vi "运维调试_总磷总氮.vi"() -> ()   [LabVIEW 2016, in "斯坦道总氮V2.lvlib"]
uses:
  <vilib>/Utility/miscctls.llb/LVPointTypeDef.ctl
  <vilib>/Plasmionique/MB Master/MB_Master/MB_Master.lvclass
  <vilib>/ptbypt/NI_PtbyPt.lvlib
panel:
  out "步骤":i32
  in  "周期设置":bool
  in  "流程写入":bool
  in  "修改系列号":bool
  out "权限等级":string
  out "总步数":i32
  out "滑动杆":u8(slide) caption="测试进度" scale=0.0..100.0
  in  "关闭心跳包":bool
  in  "仪器校准":bool
  in  "参数查询":bool
  out "简易步骤名称":string
  in  "温度曲线":bool
  in  "启动参数设置":bool
  out "固件版本号":string
  out "模块版本号":string
  out "注射器温度":sgl
  out "消解温度":sgl
  out "ADC":sgl
  out "F3":sgl format="%#.6f"
  out "F2":sgl format="%#.6f"
  out "F1":sgl format="%#.6f"
  out "F0":sgl format="%#.6f"
  out "运行状态":T1 {"数据时间:" format="%<%y/%m/%d %H:%M:%S>T"; "仪器时间:" format="%<%y/%m/%d %H:%M:%S>T"}
  in  "单选按钮":T2(radio)=enum."总氮"
  in  "布尔":bool
  out "字符串 2":string
  in  "数组":string[](array[string])
  in  "返回":bool
  in  "参数设置":bool
  out "集成报警信息":string
  in  "停止":bool
  in  "手动启动":bool
  in  "调试":bool
  out "多列列表框":i32(listbox)
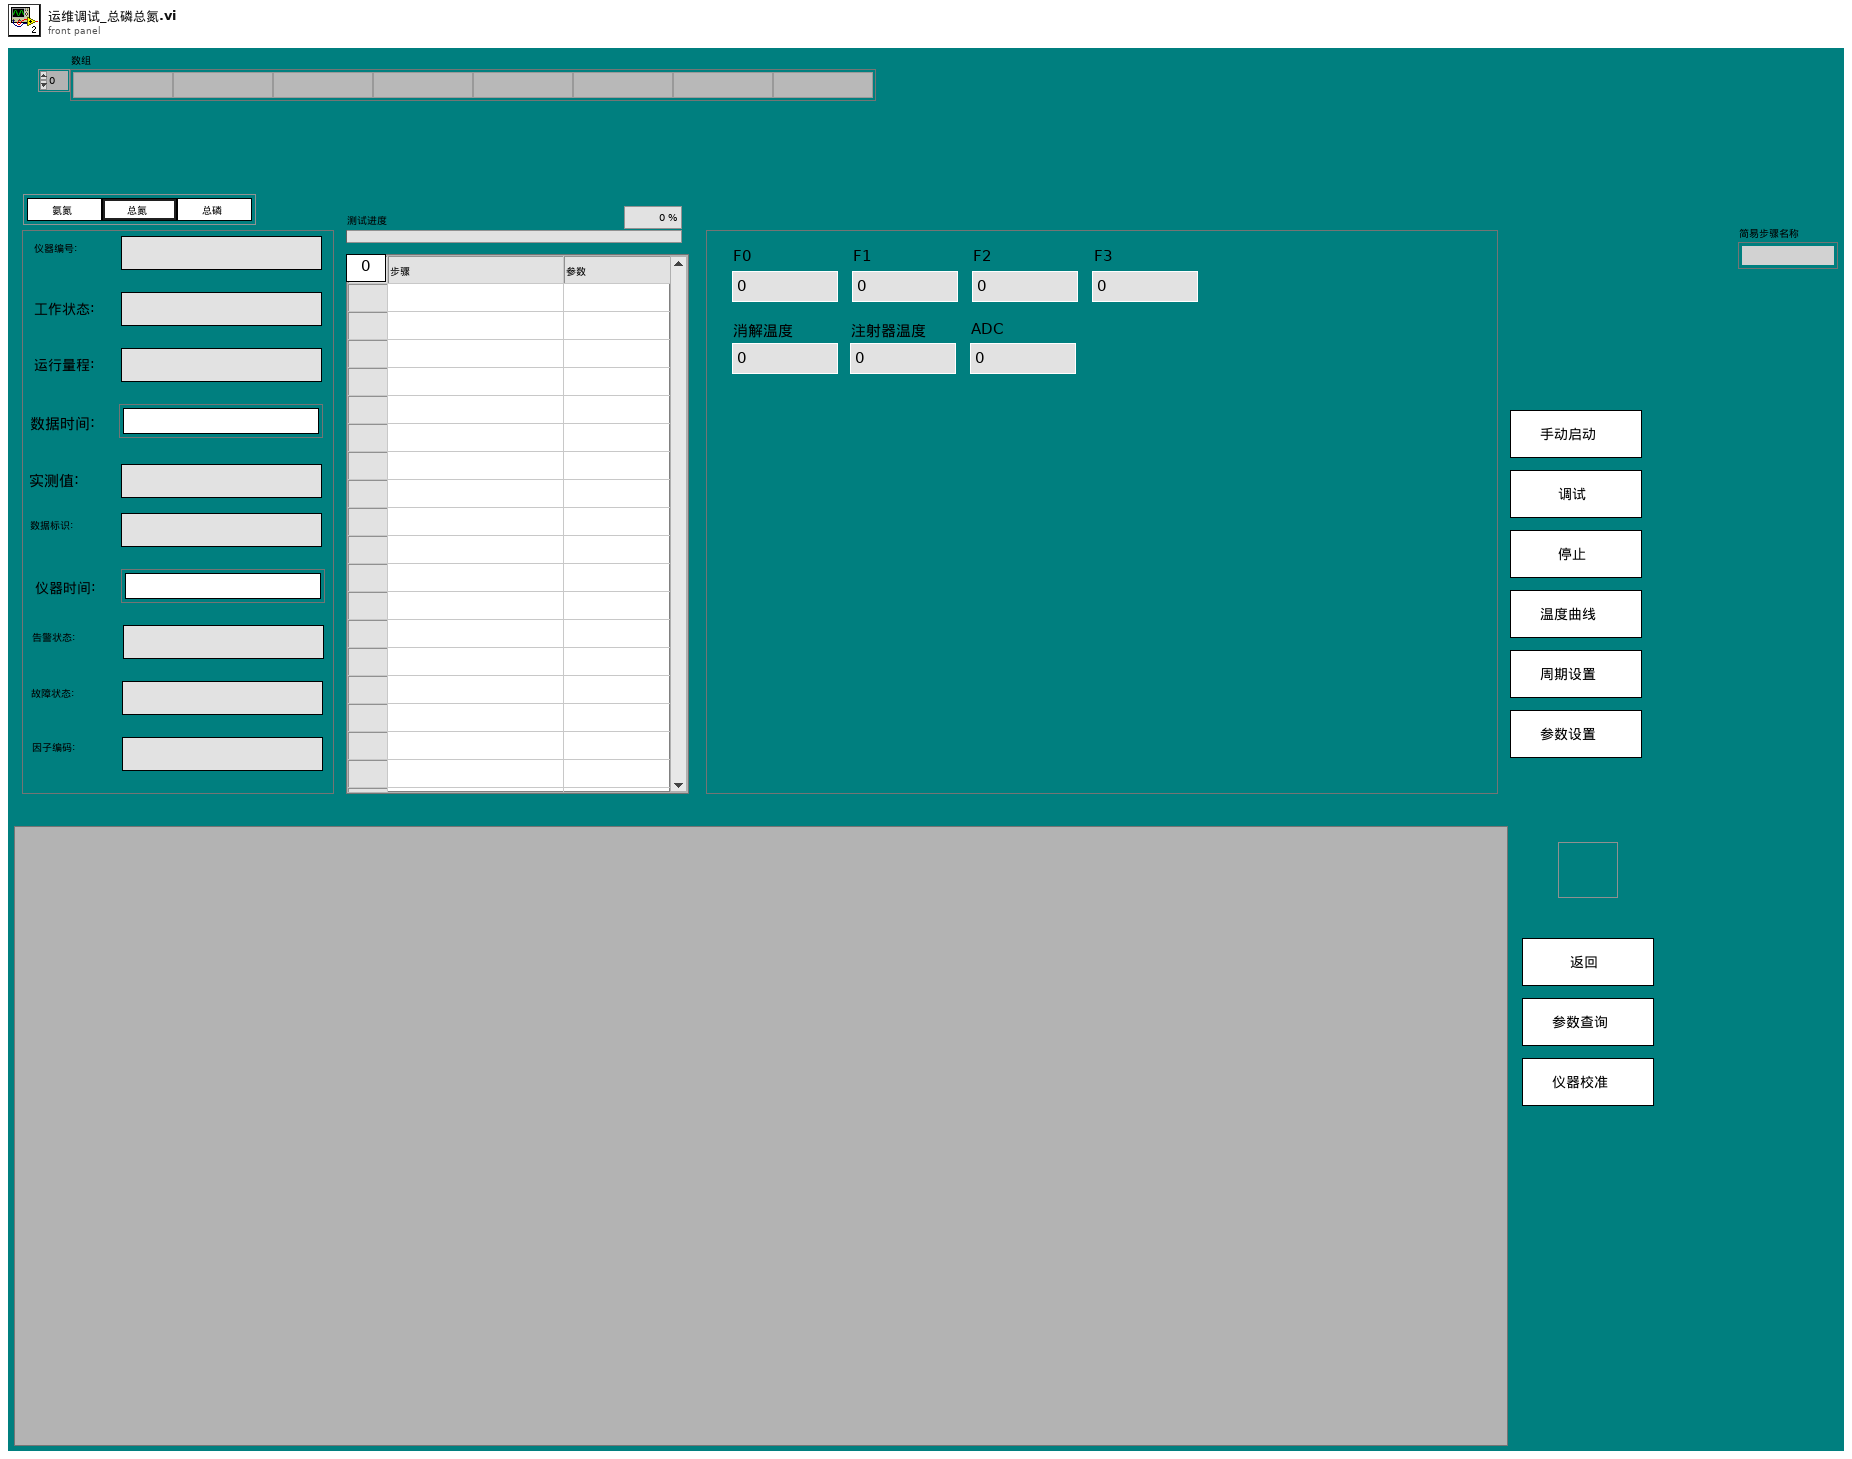
[diagram p1: front panel]
types:
  T1 = cluster{"仪器编号:":string, "工作状态:":string, "运行量程: ":string, "数据时间:":timestamp, "实测值:":string, "数据标识: ":string, "仪器时间:":timestamp, "告警状态: ":string, "故障状态:  ":string, "因子编码:":string}
  T2 = enum32{"COD", "氨氮", "总氮", "总磷", "磷酸盐", "硝氮", "亚硝氮", "硅酸盐", "硫化物"}
  T3 = cluster{"Major":u16, "Minor":u16, "Fix":u16, "Build":u16}
  T4 = typedef "LVPointTypeDef.ctl" = cluster{"Horizontal":i16, "Vertical":i16}
  T5 = cluster{"系统时间":timestamp, "工作状态":u16, "测量模式":enum16{"待机", "连续模式", "周期模式", "定点模式", "受控模式", "手动模式"}, "告警代码":u16, "故障代码":u16, "日志代码":u16, "软件版本":u16, "F0":sgl, "F1":sgl, "F2":sgl, "F3":sgl, "T":sgl, "H":sgl, "id":u16, "flowid":u16, "量程":u16, "总磷控温温度1":sgl, "营养盐控温温度2":sgl, "ADC":sgl}
  T6 = cluster{"因子编码":u32, "单位":u16, "标样参考值":sgl, "水样数据时间":timestamp, "水样实测值":sgl, "水样数据标识":string, "标样数据时间":timestamp, "标样实测值":sgl, "标样数据标识":string, "空白数据时间":timestamp, "空白实测值":sgl, "空白数据标识":string, "零点核查数据时间":timestamp, "零点核查实测值":sgl, "零点核查数据标识":string, "跨度核查数据时间":timestamp, "跨度核查实测值":sgl, "跨度核查数据标识":string, "加标回收数据时间":timestamp, "加标回收实测值":sgl, "加标回收数据标识":string, "平行样数据时间":timestamp, "平行样实测值":sgl, "平行样数据标识":string, "F0":sgl, "F1":sgl, "F2":sgl, "F3":sgl, "F4":sgl, "F5":sgl, "F6":sgl, "F7":sgl, "温度":sgl, "湿度":sgl, "X值":sgl, "fidrange":u16}[]
  T7 = cluster{"因子编码":u32, "单位":u16, "标样参考值":sgl, "水样数据时间":timestamp, "水样实测值":sgl, "水样数据标识":string, "标样数据时间":timestamp, "标样实测值":sgl, "标样数据标识":string, "空白数据时间":timestamp, "空白实测值":sgl, "空白数据标识":string, "零点核查数据时间":timestamp, "零点核查实测值":sgl, "零点核查数据标识":string, "跨度核查数据时间":timestamp, "跨度核查实测值":sgl, "跨度核查数据标识":string, "加标回收数据时间":timestamp, "加标回收实测值":sgl, "加标回收数据标识":string, "平行样数据时间":timestamp, "平行样实测值":sgl, "平行样数据标识":string, "F0":sgl, "F1":sgl, "F2":sgl, "F3":sgl, "F4":sgl, "F5":sgl, "F6":sgl, "F7":sgl, "温度":sgl, "湿度":sgl, "X值":sgl, "fidrange":u16}
  T8 = typedef "Alarm interface.lvlib/报警短信语音交互.ctl" = cluster{"参数":string, "元器件":string, "故障现象":string, "code":string, "platform_alarm_code":string, "solutionList":cluster{"reason":string, "solution":string}[]}
  T9 = typedef "TimingControl.lvlib/TimingControl.lvclass/国标控制命令.ctl" = enum16{"启动测量", "标样核查", "零点核查", "跨度核查", "空白测试", "平行样测试", "加标回收", "空白校准", "标样校准", "初始化（清洗）", "停止测试", "仪器重启", "校时", "模式设置", "测量间隔设置"}
  T10 = typedef "TimingControl.lvlib/TimingControl.lvclass/测量参数.ctl" = u16
  T11 = enum32{"Bad", "Idle", "Run top level", "Running"}
  T12 = cluster{"时间标识":timestamp, "设备":string, "日志信息":string, "流程参数":string}
  T13 = typedef "LVRowAndColumnUnsignedTypeDef.ctl" = cluster{"Row":u32, "Column":u32}
  T14 = enum16{"空闲", "水样测试", "标样核查", "零点核查", "跨度核查", "空白测试", "平行样测试", "加标回收", "空白校准", "标样校准", "初始化（清洗）"}
  T15 = cluster{"站号":u16, "量程切换":enum32{"H", "L", "AUTO"}, "控制命令":enum16{"启动测量", "标样核查", "零点核查", "跨度核查", "空白测试", "平行样测试", "加标回收", "空白校准", "标样校准", "初始化（清洗）", "停止测试", "仪器重启", "校时", "模式设置", "测量间隔设置"}, "模式设置":enum16{"待机", "连续模式", "周期模式", "定点模式", "受控模式", "手动模式"}, "测量间隔":u16}
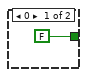
[diagram p3: hidden frame]
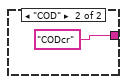
[diagram p4: hidden frame]
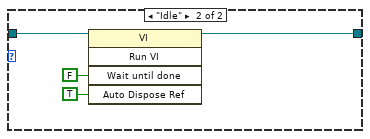
[diagram p7: hidden frame]
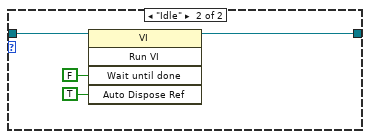
[diagram p8: hidden frame]
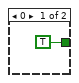
[diagram p9: hidden frame]
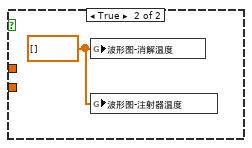
[diagram p10: hidden frame]
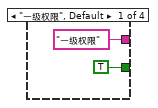
[diagram p12: hidden frame]
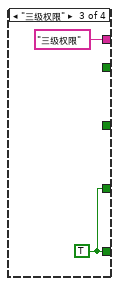
[diagram p13: hidden frame]
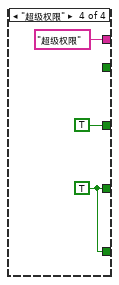
[diagram p14: hidden frame]
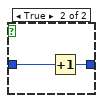
[diagram p16: hidden frame]
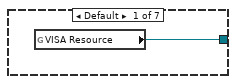
[diagram p18: hidden frame]
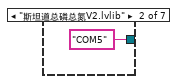
[diagram p19: hidden frame]
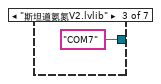
[diagram p20: hidden frame]
diagram:
  n1 = flat-sequence {
    tunnel: [w27] -> w18
    tunnel: [w26] -> w1
    tunnel: w18 -> [w38]
    tunnel: [w38] -> w4
    tunnel: w1 -> [_]
    tunnel: w4 -> [w61]
    tunnel: [w109] -> w19
    tunnel: [errorcluster {"status"=FALSE, "code"=0, "source"=""} ("错误输入（无错误）")] -> w9
    tunnel: [errorcluster {"status"=FALSE, "code"=0, "source"=""} ("错误输入（无错误）")] -> w8
    tunnel: [w106] -> w6
    tunnel: [errorcluster {"status"=FALSE, "code"=0, "source"=""} ("error out")] -> w3
    tunnel: [errorcluster {"status"=FALSE, "code"=0, "source"=""} ("错误输入（无错误）")] -> w5
    frame #0 {
      n2 = call "配置初始化.vi"() -> ("error out"=w26:errorcluster)  [unwired: 11 in]
      n3 = control-ref of="本VI"() -> (w37:refnum<vi>)
      n4 = property class="VI"(reference=w37) -> ("Library.Version"=w36:T3)  [unwired: 1 in, 2 out]
      n5 = Unbundle By Name(w36) -> ("Major"=w34:u16, "Minor"=w33:u16, "Fix"=w32:u16, "Build"=w31:u16)
      n6 = control-ref of="本VI"() -> (w28:refnum<vi>)
      n7 = Format Into String(format string="模块版本号：%d.%d.%d.%d" ("格式字符串"), w34, w33, w32, w31) -> (resulting string=→"模块版本号":string)  [unwired: 2 in, 1 out]
      n8 = property class="VI"(reference=w28) -> ("Library"=w29:refnum<vi>)  [unwired: 1 in, 2 out]
      n9 = property class="Library"(reference=w29) -> ("LocalName"=w27:string)  [unwired: 1 in, 2 out]
    }
    frame #1 {
      n10 = global read "总磷总氮断电保存全局变量.vi" "IP"() -> (w42:string)
      n11 = global read "总磷总氮断电保存全局变量.vi" "VISA Resource"() -> (w39:refnum<visa-resource-name>)
      n12 = Empty String/Path?(string/path=w42) -> (empty?=w41:bool)
      n13 = case shown="真" w41 {
        tunnel: w38 -> [_ w53]
        frame False {
        }
        frame True {
          n14 = case shown="\"斯坦道CODcrV2.lvlib\"" w53 {
            tunnel: [w54 "192.168.1.203" ("IP") "192.168.1.202" ("IP") "192.168.1.202" ("IP") "192.168.1.203" ("IP") "192.168.1.204" ("IP") "192.168.1.205" ("IP")] -> w52
            frame Default {
              n15 = global read "总磷总氮断电保存全局变量.vi" "IP"() -> (w54:string)
            }
            frame "斯坦道总磷总氮V2.lvlib" {
            }
            frame "斯坦道氨氮V2.lvlib" {
            }
            frame "斯坦道氨氮总磷V2.lvlib" {
            }
            frame "斯坦道总磷V2.lvlib" {
            }
            frame "斯坦道总氮V2.lvlib" {
            }
            frame "斯坦道CODcrV2.lvlib" {
            }
          }
          n16 = global write "总磷总氮断电保存全局变量.vi" "IP"(w52) -> ()
        }
      }
      n17 = Empty String/Path?(string/path=w39) -> (empty?=w40:bool)
      n18 = case shown="真" w40 {
        tunnel: w38 -> [_ w44]
        frame False {
        }
        frame True {
          n19 = case shown="\"斯坦道总磷V2.lvlib\"" w44 {
            tunnel: [w45 "COM5" ("IP") "COM7" ("IP") "COM7" ("IP") "COM5" ("IP") "COM10" ("IP") "COM9" ("IP")] -> w43
            frame Default {
              n20 = global read "总磷总氮断电保存全局变量.vi" "VISA Resource"() -> (w45:refnum<visa-resource-name>)
            }
            frame "斯坦道总磷总氮V2.lvlib" {
            }
            frame "斯坦道氨氮V2.lvlib" {
            }
            frame "斯坦道氨氮总磷V2.lvlib" {
            }
            frame "斯坦道总磷V2.lvlib" {
            }
            frame "斯坦道总氮V2.lvlib" {
            }
            frame "斯坦道CODcrV2.lvlib" {
            }
          }
          n21 = global write "总磷总氮断电保存全局变量.vi" "VISA Resource"(w43) -> ()
        }
      }
    }
    frame #2 {
      n22 = global read "总磷总氮断电保存全局变量.vi" "启动队列名称"() -> (w63:cluster{"String":string, "Value":u16}[])
      n23 = Empty Array?(array=w63) -> (empty?=w62:bool)
      n24 = case shown="真" w62 {
        tunnel: w61 -> [_ w64]
        frame False {
        }
        frame True {
          n25 = case shown="\"斯坦道总磷总氮V2.lvlib\"" w64 {
            frame Default {
            }
            frame "斯坦道总磷总氮V2.lvlib" {
              n26 = global write "总磷总氮断电保存全局变量.vi" "启动队列名称"(cluster{"String":string, "Value":u16}[] [{"String"="总氮", "Value"=2}, {"String"="总磷", "Value"=1}] ("启动队列名称")) -> ()
            }
            frame "斯坦道氨氮V2.lvlib" {
              n27 = global write "总磷总氮断电保存全局变量.vi" "启动队列名称"(cluster{"String":string, "Value":u16}[] [{"String"="氨氮", "Value"=3}] ("启动队列名称")) -> ()
            }
            frame "斯坦道氨氮总磷V2.lvlib" {
              n28 = global write "总磷总氮断电保存全局变量.vi" "启动队列名称"(cluster{"String":string, "Value":u16}[] [{"String"="氨氮", "Value"=3}, {"String"="总磷", "Value"=1}] ("启动队列名称")) -> ()
            }
            frame "斯坦道总磷V2.lvlib" {
              n29 = global write "总磷总氮断电保存全局变量.vi" "启动队列名称"(cluster{"String":string, "Value":u16}[] [{"String"="总磷", "Value"=1}] ("启动队列名称")) -> ()
            }
            frame "斯坦道总氮V2.lvlib" {
              n30 = global write "总磷总氮断电保存全局变量.vi" "启动队列名称"(cluster{"String":string, "Value":u16}[] [{"String"="总氮", "Value"=2}] ("启动队列名称")) -> ()
            }
            frame "斯坦道CODcrV2.lvlib" {
              n31 = global write "总磷总氮断电保存全局变量.vi" "启动队列名称"(cluster{"String":string, "Value":u16}[] [{"String"="CODcr", "Value"=22}] ("启动队列名称")) -> ()
            }
          }
        }
      }
    }
    frame #3 {
      # "初始化"
      n32 = global read "总磷总氮断电保存全局变量.vi" "流程路径"() -> (w74:path)
      n33 = global read "总磷总氮断电保存全局变量.vi" "启动队列名称"() -> (w71:cluster{"String":string, "Value":u16}[])
      n34 = call <vilib>:"Check if File or Folder Exists.vi"("path"=w74) -> ("file or folder exists?"=w78:bool)  [unwired: 8 in, 2 out]
      n35 = for {
        tunnel: w71 -> [w82] mode=indexing
        shift-right: [w81] -> w72
        shift-left: "" -> [w79]
        n36 = Unbundle By Name(w82) -> ("String"=w80:string)
        n37 = Concatenate Strings(w79, w80) -> (w81:string)
      }
      n38 = Empty String/Path?(string/path=w74) -> (empty?=w75:bool)
      n39 = Not(x=w78) -> (.not. x?=w77:bool)
      n40 = Or(x=w75, y=w77) -> (x .or. y?=w76:bool)
      n41 = global write "VAR总磷总氮全局变量.vi" "模块名称"(w72) -> ()
      n42 = case shown="真" w76 {
        frame False {
        }
        frame True {
          n43 = global read "总磷总氮断电保存全局变量.vi" "启动队列名称"() -> (w84:cluster{"String":string, "Value":u16}[])
          n44 = for {
            tunnel: w84 -> [w87] mode=indexing
            tunnel: [w86] -> w83 mode=indexing
            n45 = Unbundle By Name(w87) -> ("String"=w86:string)
          }
          n46 = call "获取默认流程路径.vi"("参数"=w83) -> ("路径"=w85:path)  [unwired: 10 in]
          n47 = global write "总磷总氮断电保存全局变量.vi" "流程路径"(w85) -> ()
        }
      }
    }
    frame #4 {
      n48 = vi-ref "总磷总氮通讯.vi"() -> (w88:refnum<vi>)
      n49 = vi-ref "总磷总氮测量数据储存.vi"() -> (w96:refnum<vi>)
      n50 = property class="VI"(reference=w88) -> ("Name"=w89:string)  [unwired: 1 in, 2 out]
      n51 = property class="VI"(reference=w96) -> ("Name"=w103:string)  [unwired: 1 in, 2 out]
      n52 = Open VI Reference(type specifier VI Refnum (for type only)=refnum<vi> refnum, vi path=w89, options=128 ("选项")) -> (vi reference=w91:refnum<vi>, error out=w93:errorcluster)  [unwired: 3 in]
      n53 = call-by-ref "开始异步调用"(reference=w91, error in=w93) -> (reference out=w95:refnum<vi>, error out=w94:errorcluster)  [unwired: 12 in]
      n54 = Open VI Reference(type specifier VI Refnum (for type only)=refnum<vi> refnum, vi path=w103, options=128 ("选项")) -> (vi reference=w101:refnum<vi>, error out=w99:errorcluster)  [unwired: 3 in]
      n55 = Close Reference(reference=w95, error in (no error)=w94) -> ()  [unwired: 1 out]
      n56 = call-by-ref "开始异步调用"(reference=w101, error in=w99) -> (reference out=w97:refnum<vi>, error out=w98:errorcluster)  [unwired: 12 in]
      n57 = Close Reference(reference=w97, error in (no error)=w98) -> ()  [unwired: 1 out]
    }
    frame #5 {
      n58 = call "配置文件路径.vi"() -> ("appended path"=w106:path)  [unwired: 11 in]
      n59 = call "设置模块队列名.vi"() -> ("Msg"=w109:string)  [unwired: 5 in]
    }
  }
  n60 = flat-sequence {
    frame #0 {
      n61 = property on="窗格" class="Pane"("Origin"=T4 {"Horizontal"=0, "Vertical"=0} ("原点")) -> ()  [unwired: 2 in, 2 out]
    }
  }
  n62 = while {
    shift-right: [w121] -> _
    shift-left: _ -> [w119]
    stop <- FALSE stop-if-true
    n63 = global write "VAR总磷总氮全局变量.vi" "最近一次工作状态"(w119) -> ()
    n64 = global read "VAR总磷总氮全局变量.vi" "状态告警区"() -> (w139:T5)
    n65 = global read "VAR总磷总氮全局变量.vi" "通讯状态"() -> (w150:bool)
    n66 = Wait (ms)(milliseconds to wait=u32 1000 ("等待时间（毫秒）")) -> ()  [unwired: 1 out]
    n67 = case shown="\"氨氮\"" "单选按钮" {
      tunnel: [22 3 2 1 4 5 6 7 8] -> w113
      frame "COD", Default {
      }
      frame "氨氮" {
      }
      frame "总氮" {
      }
      frame "总磷" {
      }
      frame "磷酸盐" {
      }
      frame "硝氮" {
      }
      frame "亚硝氮" {
      }
      frame "硅酸盐" {
      }
      frame "硫化物" {
      }
    }
    n68 = Unbundle By Name(w139) -> ("id"=w138:u16, "工作状态"=w135:u16)
    n69 = case shown="真" w150 {
      tunnel: ["通讯异常" ("集成报警信息") w244] -> w149
      frame False {
      }
      frame True {
        n70 = global read "VAR总磷总氮全局变量.vi" "状态告警区"() -> (w250:T5)
        n71 = Unbundle By Name(w250) -> ("工作状态"=w249:u16)
        n72 = feedback #1(0) -> (w247:i32)
        n73 = case shown="0" w249 {
          tunnel: w247 -> [_ w252]
          tunnel: [_ w251] -> w245
          frame 0 {
          }
          frame Default {
            n74 = Increment(x=w252) -> (x+1=w251:i32)
          }
        }
        n75 = feedback-in #1(w245) -> ()
        n76 = global read "VAR总磷总氮全局变量.vi" "测量状态"() -> (w243:string)
        n77 = Format Into String(format string="工作计时: %d 秒" ("格式字符串"), initial string=w243, w245) -> (resulting string=w244:string)  [unwired: 1 in, 1 out]
      }
    }
    "集成报警信息" <- w149
    n78 = global read "VAR总磷总氮全局变量.vi" "测量数据区数组"() -> (w124:T6)
    n79 = case shown="1, 默认" w135 {
      tunnel: w138 -> [_ w195]
      frame 0 {
      }
      frame 1, Default {
        n80 = case shown="3, 92" w195 {
          frame 0, Default {
          }
          frame 1, 131 {
            n81 = local write "单选按钮"(T2."总磷" ("单选按钮")) -> ()
          }
          frame 2, 76 {
            n82 = local write "单选按钮"(T2."总氮" ("单选按钮")) -> ()
          }
          frame 22 {
            n83 = local write "单选按钮"(T2."COD" ("单选按钮")) -> ()
          }
          frame 3, 92 {
            n84 = local write "单选按钮"(T2."氨氮" ("单选按钮")) -> ()
          }
          frame 4 {
            n85 = local write "单选按钮"(T2."磷酸盐" ("单选按钮")) -> ()
          }
          frame 5 {
            n86 = local write "单选按钮"(T2."硝氮" ("单选按钮")) -> ()
          }
          frame 6 {
            n87 = local write "单选按钮"(T2."亚硝氮" ("单选按钮")) -> ()
          }
          frame 7 {
            n88 = local write "单选按钮"(T2."硅酸盐" ("单选按钮")) -> ()
          }
          frame 8 {
            n89 = local write "单选按钮"(T2."硫化物" ("单选按钮")) -> ()
          }
        }
      }
    }
    n90 = call "id参数转换.vi"("id"=w113) -> ("数组资源索引"=w111:i32)  [unwired: 9 in, 1 out]
    n91 = Index Array(array=w124, index=w111) -> (element=w123:T7)
    n92 = case shown="0, 默认" w119 {
      tunnel: [w164 w170 w174 w178 w182 w186 w190 w194] -> w134
      tunnel: [w162 w169 w173 w177 w180 w185 w189 w193] -> w129
      tunnel: [w165 w168 w172 w176 w179 w184 w188 w192] -> w127
      tunnel: w123 -> [_ w167 w171 w175 w181 w183 w187 w191]
      frame 0, Default {
        n93 = local read "运行状态"() -> (w166:T1)
        n94 = Unbundle By Name(w166) -> ("数据时间:"=w164:timestamp, "实测值:"=w163:string, "数据标识:"=w165:string)
        n95 = Fract/Exp String To Number(string=w163) -> (number=w162:dbl)  [unwired: 3 in, 1 out]
      }
      frame 1 {
        n96 = Unbundle By Name(w167) -> ("水样数据时间"=w170:timestamp, "水样实测值"=w169:sgl, "水样数据标识"=w168:string)
      }
      frame 2, 9 {
        n97 = Unbundle By Name(w171) -> ("标样数据时间"=w174:timestamp, "标样实测值"=w173:sgl, "标样数据标识"=w172:string)
      }
      frame 3 {
        n98 = Unbundle By Name(w175) -> ("零点核查数据时间"=w178:timestamp, "零点核查实测值"=w177:sgl, "零点核查数据标识"=w176:string)
      }
      frame 4 {
        n99 = Unbundle By Name(w181) -> ("跨度核查数据时间"=w182:timestamp, "跨度核查实测值"=w180:sgl, "跨度核查数据标识"=w179:string)
      }
      frame 7 {
        n100 = Unbundle By Name(w183) -> ("加标回收数据时间"=w186:timestamp, "加标回收实测值"=w185:sgl, "加标回收数据标识"=w184:string)
      }
      frame 5, 8 {
        n101 = Unbundle By Name(w187) -> ("空白数据时间"=w190:timestamp, "空白实测值"=w189:sgl, "空白数据标识"=w188:string)
      }
      frame 6 {
        n102 = Unbundle By Name(w191) -> ("平行样数据时间"=w194:timestamp, "平行样实测值"=w193:sgl, "平行样数据标识"=w192:string)
      }
    }
    n103 = Unbundle By Name(w123) -> ("因子编码"=w125:u32)
    n104 = global read "VAR总磷总氮全局变量.vi" "状态告警区"() -> (w148:T5)
    n105 = Unbundle By Name(w148) -> ("flowid"=w118:u16, "系统时间"=w144:timestamp, "工作状态"=w143:u16, "告警代码"=w137:u16, "故障代码"=w136:u16, "量程"=w142:u16)
    n106 = First Call?() -> (First Call?: T/F=w112:bool)
    n107 = case shown="10" w143 {
      selector: w143 -> [w209 _ w215 w219 w222 w224 w226 w228 w230 w232 w234 w236 w238 w241]
      tunnel: [w210 "空闲" ("工作状态") "水样测量" ("工作状态") w218 "零点核查" ("工作状态") "跨度核查" ("工作状态") "空白测试" ("工作状态") "平行样测试" ("工作状态") "加标回收" ("工作状态") "空白校准" ("工作状态") "标样校准" ("工作状态") "初始化" ("工作状态") "单步调试" ("工作状态") w240] -> w120
      tunnel: [w208 w213 w215 w219 w222 w224 w226 w228 w230 w232 w234 w236 w238 w241] -> w121
      tunnel: w119 -> [w208 w213 _ _ _ _ _ _ _ _ _ _ _ _]
      tunnel: w118 -> [_ _ _ w217 _ _ _ _ _ _ _ _ _ _]
      frame Default {
        n108 = Format Into String(format string="%d" ("格式字符串"), initial string="未知" ("工作状态"), w209) -> (resulting string=w210:string)  [unwired: 1 in, 1 out]
      }
      frame 0 {
      }
      frame 1 {
      }
      frame 2 {
        n109 = case shown="0, 默认" w217 {
          tunnel: ["标样核查" ("工作状态") "快捷测试" ("工作状态")] -> w218
          frame 0, Default {
          }
          frame 5 {
          }
        }
      }
      frame 3 {
      }
      frame 4 {
      }
      frame 5 {
      }
      frame 6 {
      }
      frame 7 {
      }
      frame 8 {
      }
      frame 9 {
      }
      frame 10 {
      }
      frame 254 {
      }
      frame 255 {
        n110 = local read "简易步骤名称"() -> (w240:string)
      }
    }
    n111 = call "告警码字段定义.vi"("id"=w113, "首次调用？"=w112, "告警代码"=w137) -> ("报警"=w117:T8)  [unwired: 8 in]
    n112 = call "故障码字段定义.vi"("id"=w113, "首次调用？"=w112, "故障代码"=w136) -> ("报警"=w115:T8)  [unwired: 8 in]
    n113 = Unbundle By Name(w117) -> ("故障现象"=w116:string)
    n114 = Unbundle By Name(w115) -> ("故障现象"=w114:string)
    n115 = case shown="1" w142 {
      tunnel: ["" ("字符串") "低量程 " ("字符串") "高量程 " ("字符串")] -> w141
      frame Default {
      }
      frame 0 {
      }
      frame 1 {
      }
    }
    n116 = Number To Fractional String(number=w129, precision (6)=i16 4 ("精度(6)")) -> (F-format string=w131:string)  [unwired: 2 in]
    n117 = Concatenate Strings(w131, " " ("字符串"), "mg/L" ("字符串")) -> (w128:string)
    n118 = global read "VAR总磷总氮全局变量.vi" "序列号"() -> (w145:string)
    n119 = Format Into String(format string="w%05d" ("格式字符串"), w125) -> (resulting string=w140:string)  [unwired: 2 in, 1 out]
    n120 = global write "VAR总磷总氮全局变量.vi" "工作状态:"(w120) -> ()
    n121 = Bundle By Name(cluster=T1 {"仪器编号:"="", "工作状态:"="", "运行量程: "="", "数据时间:"=timestamp(0 s since 1904-01-01), "实测值:"="", "数据标识: "="", "仪器时间:"=timestamp(0 s since 1904-01-01), "告警状态: "="", "故障状态:  "="", "因子编码:"=""} ("运行状态"), "仪器编号:"=w145, "仪器时间:"=w144, "工作状态:"=w120, "告警状态:"=w116, "故障状态:"=w114, "运行量程:"=w141, "数据时间:"=w134, "实测值:"=w128, "数据标识:"=w127, "因子编码:"=w140) -> (→"运行状态":T1)
  }
  n122 = while {
    shift-right: [w263] -> _
    shift-left: u32 0 ("y") -> [w265]
    stop <- FALSE stop-if-true
    # "密码权限"
    n123 = global read "VAR总磷总氮全局变量.vi" "权限等级"() -> (w260:enum16{"一级权限", "二级权限", "三级权限", "超级权限"})
    n124 = case shown="假" "布尔" {
      tunnel: w265 -> [_ w278]
      tunnel: [_ w277] -> w263
      frame False {
      }
      frame True {
        n125 = Increment(x=w278) -> (x+1=w277:u32)
      }
    }
    n126 = Wait (ms)(milliseconds to wait=u32 1000 ("等待时间（毫秒）")) -> ()  [unwired: 1 out]
    n127 = case shown="\"二级权限\"" w260 {
      tunnel: [_ TRUE w272 w275] -> w253
      tunnel: [_ _ w272 w275] -> w254
      tunnel: [_ _ _ TRUE] -> w259
      tunnel: [TRUE _ _ _] -> w257
      tunnel: ["一级权限" "二级权限" "三级权限" "超级权限"] -> w255
      frame "一级权限", Default {
      }
      frame "二级权限" {
      }
      frame "三级权限" {
        w272 = TRUE
      }
      frame "超级权限" {
        w275 = TRUE
      }
    }
    "权限等级" <- w255
    n128 = property on="关闭心跳包" class="Bool (严格)"("Visible"=w259) -> ()  [unwired: 2 in, 2 out]
    n129 = property on="流程写入" class="Bool"("Visible"=w253) -> ()  [unwired: 2 in, 2 out]
    n130 = property on="修改系列号" class="Bool"("Visible"=w254) -> ()  [unwired: 2 in, 2 out]
    n131 = property on="启动参数设置" class="Bool"("Visible"=w254) -> ()  [unwired: 2 in, 2 out]
    n132 = Greater Or Equal?(x=w263, y=u32 3600) -> (x >= y?=w261:bool)
    n133 = Not(x=w257) -> (.not. x?=w256:bool)
    n134 = property on="布尔" class="Bool (严格)"("Value"=w256) -> ()  [unwired: 2 in, 2 out]
    n135 = case shown="真" w261 {
      frame False {
      }
      frame True {
        n136 = global write "VAR总磷总氮全局变量.vi" "权限等级"(enum16{"一级权限", "二级权限", "三级权限", "超级权限"}."一级权限" ("权限等级")) -> ()
      }
    }
  }
  n137 = while {
    shift-right: [w283] -> _
    shift-left: 0 -> [w284]
    stop <- FALSE stop-if-true
    n138 = global read "VAR总磷总氮全局变量.vi" "心跳包打开状态"() -> (w279:bool)
    n139 = Wait (ms)(milliseconds to wait=u32 1000 ("等待时间（毫秒）")) -> ()  [unwired: 1 out]
    n140 = case shown="假" w279 {
      tunnel: w284 -> [w288 _]
      tunnel: [w287 _] -> w283
      frame False {
        n141 = Increment(x=w288) -> (x+1=w287:i32)
      }
      frame True {
      }
    }
    n142 = Greater Or Equal?(x=w283, y=3600) -> (x >= y?=w281:bool)
    n143 = case shown="真" w281 {
      frame False {
      }
      frame True {
        w286 = FALSE ("关闭心跳包")
        n144 = local write "关闭心跳包"(w286) -> ()
        n145 = global write "VAR总磷总氮全局变量.vi" "升级固件关闭心跳包"(w286) -> ()
      }
    }
  }
  n146 = while {
    shift-right: [w290] -> _
    shift-left: TRUE -> [w289]
    stop <- FALSE stop-if-true
    n147 = global read "VAR总磷总氮全局变量.vi" "状态告警区"() -> (w294:T5)
    n148 = Wait (ms)(milliseconds to wait=u32 1000 ("等待时间（毫秒）")) -> ()  [unwired: 1 out]
    n149 = Unbundle By Name(w294) -> ("工作状态"=w291:u16, "总磷控温温度1"=w293:sgl, "营养盐控温温度2"=w292:sgl)
    n150 = case shown="1, 默认" w291 {
      tunnel: w293 -> [_ w300]
      tunnel: w292 -> [_ w299]
      tunnel: [TRUE _] -> w290
      tunnel: w289 -> [_ w298]
      frame 0 {
      }
      frame 1, Default {
        n151 = case shown="假" w298 {
          tunnel: w300 -> [w306 _]
          tunnel: w299 -> [w305 _]
          frame False {
            n152 = global read "VAR总磷总氮全局变量.vi" "波形图-消解温度"() -> (w304:dbl[])
            n153 = global read "VAR总磷总氮全局变量.vi" "波形图-注射器温度"() -> (w303:dbl[])
            n154 = Insert Into Array(array=w304, new element=w306) -> (w302:dbl[])  [unwired: 1 in]
            n155 = Insert Into Array(array=w303, new element=w305) -> (w301:dbl[])  [unwired: 1 in]
            n156 = global write "VAR总磷总氮全局变量.vi" "波形图-消解温度"(w302) -> ()
            n157 = global write "VAR总磷总氮全局变量.vi" "波形图-注射器温度"(w301) -> ()
          }
          frame True {
            w307 = dbl[] [] ("波形图-消解温度")
            n158 = global write "VAR总磷总氮全局变量.vi" "波形图-消解温度"(w307) -> ()
            n159 = global write "VAR总磷总氮全局变量.vi" "波形图-注射器温度"(w307) -> ()
          }
        }
      }
    }
  }
  n160 = while {
    shift-right: [w308] -> _
    shift-left: _ -> [w313]
    tunnel: w6 -> [w311]
    stop <- FALSE stop-if-true
    n161 = File/Directory Info(path=w311) -> (last mod=w308:timestamp, error out=w309:errorcluster)  [unwired: 1 in, 5 out]
    n162 = Wait (ms)(milliseconds to wait=u32 1000 ("等待时间（毫秒）")) -> ()  [unwired: 1 out]
    n163 = Not Equal?(x=w313, y=w308) -> (x != y?=w312:bool)
    n164 = case shown="真" w312 {
      tunnel: [_ w315] -> _
      tunnel: w309 -> [_ _]
      frame False {
      }
      frame True {
        n165 = call "配置读取.vi"() -> ("error out"=w315:errorcluster)  [unwired: 11 in]
      }
    }
  }
  n166 = flat-sequence {
    tunnel: w3 -> [_]
    frame #0 {
      n167 = control-ref of="周期设置"() -> (w318:refnum<vi>)
      n168 = call "New TimingControl.vi"("Reference"=w318) -> ("error out"=w319:errorcluster, "TimingControl out"=w320:refnum<class "TimingControl.lvclass">)  [unwired: 9 in]
      n169 = call "taskqueue ref.vi"() -> ("队列输出"=w321:refnum<queue>)  [unwired: 10 in, 1 out]
      n170 = while {
        tunnel: w321 -> [w333]
        shift-right: [w324] -> w317
        shift-left: w320 -> [w328]
        shift-right: [w326] -> w316
        shift-left: w319 -> [w327]
        stop <- FALSE stop-if-true
        n171 = Wait (ms)(milliseconds to wait=u32 500 ("等待时间（毫秒）")) -> ()  [unwired: 1 out]
        n172 = global read "VAR总磷总氮全局变量.vi" "状态告警区"() -> (w335:T5)
        n173 = Unbundle By Name(w335) -> ("工作状态"=w334:u16, "系统时间"=w322:timestamp)
        n174 = case shown="1, 默认" w334 {
          tunnel: [FALSE TRUE] -> w323
          frame 0 {
          }
          frame 1, Default {
          }
        }
        n175 = property class="TimingControl"(reference=w328, error in=w327, "Properties:仪器时间"=w322, "Properties:仪器运行状态"=w323) -> (reference out=w324:refnum<class "TimingControl.lvclass">, error out=w326:errorcluster, "Properties:命令输出"=w325:cluster{"启动":bool, "控制命令":T9, "测量参数":T10})
        n176 = Unbundle By Name(w325) -> ("启动"=w331:bool, "控制命令"=w332:T9)
        n177 = call <vilib>:"Boolean Crossing PtByPt.vi"("direction"=enum16{"either", "false-true", "true-false"}."false-true", "input"=w331) -> ("crossing"=w329:bool)  [unwired: 1 in]
        n178 = case shown="真" w329 {
          tunnel: w333 -> [_ w339]
          tunnel: w332 -> [_ w338]
          frame False {
          }
          frame True {
            n179 = Enqueue Element(queue=w339, element=w338) -> ()  [unwired: 2 in, 3 out]
          }
        }
      }
      n180 = call "task.vi"() -> ()  [unwired: 12 in]
      n181 = call "Close TimingControl.vi"("error in (no error)"=w316, "TimingControl in"=w317) -> ()  [unwired: 9 in, 1 out]
    }
  }
  n182 = while {
    tunnel: w3 -> [_]
    stop <- FALSE stop-if-true
    n183 = flat-sequence {
      frame #0 {
        n184 = global read "总磷总氮断电保存全局变量.vi" "启动队列名称"() -> (w346:cluster{"String":string, "Value":u16}[])
        n185 = global read "总磷总氮断电保存全局变量.vi" "启动队列名称"() -> (w344:cluster{"String":string, "Value":u16}[])
        n186 = for {
          tunnel: w344 -> [w354] mode=indexing
          tunnel: [w353] -> w345 mode=indexing
          n187 = Unbundle By Name(w354) -> ("String"=w353:string)
        }
        n188 = for {
          tunnel: w346 -> [w352] mode=indexing
          shift-right: [w351] -> w347
          shift-left: "" -> [w349]
          n189 = Unbundle By Name(w352) -> ("String"=w350:string)
          n190 = Concatenate Strings(w349, w350) -> (w351:string)
        }
        n191 = property on="单选按钮" class="RadioBtnsControl (严格)"() -> ("Controls[]"=w343:refnum<vi>[])  [unwired: 2 in, 2 out]
        n192 = for {
          tunnel: w343 -> [w362] mode=indexing
          tunnel: w345 -> [w361]
          n193 = property class="Ctl"(reference=w362) -> (reference out=w360:refnum<vi>, "Label.Text"=w356:string)  [unwired: 1 in, 1 out]
          n194 = case shown="默认" w356 {
            selector: w356 -> [w363 _]
            tunnel: [w363 "CODcr"] -> w355
            frame Default {
            }
            frame "COD" {
            }
          }
          n195 = Search 1D Array(1D array=w361, element=w355) -> (index of element=w359:i32)  [unwired: 1 in]
          n196 = Not Equal?(x=w359, y=-1) -> (x != y?=w357:bool)
          n197 = property class="Ctl"(reference=w360, "Visible"=w357) -> ()  [unwired: 1 in, 2 out]
        }
        n198 = global write "VAR总磷总氮全局变量.vi" "模块名称"(w347) -> ()
      }
      frame #1 {
        n199 = Wait (ms)(milliseconds to wait=u32 1000 ("等待时间（毫秒）")) -> ()  [unwired: 1 out]
      }
    }
  }
  n200 = call "时间延迟"("error in (no error)"=w5) -> ("error out"=w25:errorcluster)  [unwired: 10 in]
  n201 = vi-ref "校准设置页.vi"() -> (w13:refnum<vi>)
  n202 = vi-ref "参数设置页.vi"() -> (w17:refnum<vi>)
  n203 = property class="VI"(reference=w13, error in=w8) -> (reference out=w11:refnum<vi>, "Exec.State"=w12:T11)  [unwired: 1 out]
  n204 = property class="VI"(reference=w17, error in=w9) -> (reference out=w15:refnum<vi>, "Exec.State"=w16:T11)  [unwired: 1 out]
  n205 = while {
    tunnel: w25 -> [_]
    stop <- FALSE stop-if-true
    n206 = Wait (ms)(milliseconds to wait=u32 1000 ("等待时间（毫秒）")) -> ()  [unwired: 1 out]
    n207 = global read "VAR总磷总氮全局变量.vi" "状态告警区"() -> (w396:T5)
    n208 = global read "VAR总磷总氮全局变量.vi" "状态告警区"() -> (w397:T5)
    n209 = global read "VAR总磷总氮全局变量.vi" "状态告警区"() -> (w395:T5)
    n210 = global read "VAR总磷总氮全局变量.vi" "状态告警区"() -> (w393:T5)
    n211 = Unbundle By Name(w397) -> ("id"=w376:u16, "flowid"=w375:u16, "量程"=w374:u16, "工作状态"=w378:u16, "F0"=→"F0":sgl, "F1"=→"F1":sgl, "F2"=→"F2":sgl, "F3"=→"F3":sgl, "ADC"=→"ADC":sgl, "总磷控温温度1"=→"消解温度":sgl, "营养盐控温温度2"=→"注射器温度":sgl)  [unwired: 1 out]
    n212 = Unbundle By Name(w393) -> ("日志代码"=w392:u16)
    n213 = Unbundle By Name(w396) -> ("日志代码"=w372:u16)
    n214 = Unbundle By Name(w395) -> ("flowid"=w369:u16, "工作状态"=w388:u16, "id"=w389:u16)
    n215 = case shown="0" w388 {
      frame 0 {
        n216 = local write "数组"(string[] [] ("数组")) -> ()
      }
      frame 1, Default {
      }
    }
    n217 = feedback-in #2(w372) -> ()
    n218 = feedback #2(w372) -> (w399:u16)
    n219 = feedback #3(w392) -> (w394:u16)
    n220 = feedback-in #3(w392) -> ()
    n221 = Not Equal To 0?(x=w388) -> (x != 0?=w367:bool)
    n222 = property on="总步数" class="DigNum (严格)"() -> ("Value"=w373:i32)  [unwired: 2 in, 2 out]
    n223 = Subtract(x=w372, y=1) -> (x-y=→"多列列表框" →"步骤":i32)
    n224 = Divide(x=w372, y=w373) -> (x/y=w371:dbl)
    n225 = Not Equal?(x=w372, y=w399) -> (x != y?=w398:bool)
    n226 = Not Equal?(x=w392, y=w394) -> (x != y?=w391:bool)
    n227 = call <vilib>:"Boolean Crossing PtByPt.vi"("direction"=enum16{"either", "false-true", "true-false"}."either", "input"=w367) -> ("crossing"=w386:bool)  [unwired: 1 in]
    n228 = Bundle("id"=w376, "flowid"=w375, "量程"=w374) -> (w377:cluster{"id":u16, "flowid":u16, "量程":u16})  [unwired: 1 in]
    n229 = case shown="真" w398 {
      tunnel: w372 -> [_ w547]
      frame False {
      }
      frame True {
        n230 = Subtract(x=w547, y=1) -> (x-y=w545:i32)
        n231 = Subtract(x=w545, y=5) -> (x-y=w549:i32)
        n232 = Greater Or Equal To 0?(x=w549) -> (x >= 0?=w548:bool)
        n233 = Select(t=w549, s=w548, f=0) -> (s? t:f=w550:i32)
        n234 = property on="多列列表框" class="MCListbox (严格)"() -> (error out=w553:errorcluster, "TopLeft"=w554:T13)  [unwired: 2 in, 1 out]
        n235 = Bundle By Name(cluster=w554, "Row"=w550) -> (w555:T13)
        n236 = property on="多列列表框" class="MCListbox (严格)"(error in=w553, "TopLeft"=w555) -> ()  [unwired: 1 in, 2 out]
      }
    }
    n237 = while {
      tunnel: w377 -> [w531]
      shift-right: [w527] -> _
      shift-left: _ -> [w528]
      shift-right: [w520] -> _
      shift-left: _ -> [w529]
      shift-right: [w521] -> _
      shift-left: _ -> [w526]
      tunnel: w378 -> [w518]
      shift-right: [w518] -> _
      shift-left: _ -> [w524]
      stop <- TRUE stop-if-true
      n238 = Not Equal?(x=w524, y=w518) -> (x != y?=w523:bool)
      n239 = global read "总磷总氮断电保存全局变量.vi" "流程路径"() -> (w521:path)
      n240 = Not Equal?(x=w526, y=w521) -> (x != y?=w522:bool)
      n241 = Compound Arithmetic op=OR ("复合运算")(w522, w523) -> (w525:bool)
      n242 = case shown="真" w525 {
        tunnel: [w533 w543] -> w520
        tunnel: [w532 w542] -> w527
        tunnel: w531 -> [_ w537]
        tunnel: w529 -> [w533 _]
        tunnel: w528 -> [w532 _]
        tunnel: w521 -> [_ w536]
        tunnel: w518 -> [_ w535]
        frame False {
        }
        frame True {
          n243 = call "斯坦道XML解析.vi"("工作状态"=w535, "添加的路径"=w536, "参数簇"=w537) -> ("简易步骤名称"=→"简易步骤名称":string, "步骤时间"=w538:string[], "步骤名"=w540:string[])  [unwired: 6 in]
          n244 = for {
            tunnel: w540 -> [_] mode=indexing
            tunnel: [w544] -> w541 mode=indexing
            i -> [w544]
          }
          n245 = Build Array(w540, w538) -> (w539:string[][])
          n246 = Transpose 2D Array(2D array=w539) -> (transposed array=w542:string[][])
          n247 = Number To Decimal String(number=w541) -> (decimal integer string=w543:string[])  [unwired: 1 in]
        }
      }
      n248 = property on="多列列表框" class="MCListbox (严格)"("ItemNames"=w527, "RowHdrs[]"=w520) -> ()  [unwired: 2 in, 2 out]
      n249 = Array Size(array=w520) -> (size(s)=→"总步数":i32)
    }
    n250 = case shown="真" w386 {
      tunnel: w389 -> [_ w423]
      tunnel: w369 -> [_ w410]
      tunnel: w367 -> [_ w408]
      frame False {
      }
      frame True {
        n251 = global read "VAR总磷总氮全局变量.vi" "最近一次工作状态"() -> (w409:u16)
        n252 = case shown="2" w409 {
          selector: w409 -> [w429 _ _ _ _ _ _ _ _ _ _ _]
          tunnel: [w428 "【水样测试】" ("字符串") w432 "【零点核查】" ("字符串") "【跨度核查】" ("字符串") "【空白测试】" ("字符串") "【平行样测试】" ("字符串") "【加标回收】" ("字符串") "【空白校准】" ("字符串") "【标样校准】" ("字符串") "【单步调试】" ("字符串") "【简易流程】" ("字符串")] -> w404
          tunnel: w410 -> [_ _ w431 _ _ _ _ _ _ _ _ _]
          frame 0, Default {
            n253 = Number To Decimal String(number=w429) -> (decimal integer string=w428:string)  [unwired: 1 in]
          }
          frame 1 {
          }
          frame 2 {
            n254 = case shown="5" w431 {
              tunnel: ["【标样核查】" ("字符串") "【快捷测试】" ("字符串")] -> w432
              frame 0, Default {
              }
              frame 5 {
              }
            }
          }
          frame 3 {
          }
          frame 4 {
          }
          frame 5 {
          }
          frame 6 {
          }
          frame 7 {
          }
          frame 8 {
          }
          frame 9 {
          }
          frame 254 {
          }
          frame 255 {
          }
        }
        n255 = global read "VAR总磷总氮全局变量.vi" "状态告警区"() -> (w421:T5)
        n256 = Concatenate Strings("<<" ("字符串"), w404, "启动" ("字符串")) -> (w405:string)
        n257 = Concatenate Strings(w404, "停止" ("字符串"), ">>" ("字符串")) -> (w403:string)
        n258 = Unbundle By Name(w421) -> ("F0"=w420:sgl, "F1"=w419:sgl, "F2"=w418:sgl, "F3"=w417:sgl, "id"=w416:u16, "flowid"=w415:u16, "量程"=w414:u16)
        n259 = Format Into String(format string="F0=%#f,F1=%#f,F2=%#f,F3=%#f,Flow=%d-%-d-%-d" ("格式字符串"), w420, w419, w418, w417, w416, w415, w414) -> (resulting string=w412:string)  [unwired: 2 in, 1 out]
        n260 = Select(t=w405, s=w408, f=w403) -> (s? t:f=w402:string)
        n261 = call "id参数转换.vi"("id"=w423) -> ("table输出"=w422:string)  [unwired: 9 in, 1 out]
        n262 = Get Date/Time In Seconds() -> (seconds since 1Jan1904=w426:timestamp)
        n263 = Bundle By Name(cluster=T12 {"时间标识"=timestamp(0 s since 1904-01-01), "设备"="", "日志信息"="", "流程参数"=""} ("data in"), "时间标识"=w426, "设备"=w422, "日志信息"=w402, "流程参数"=w412) -> (w425:T12)
        n264 = call "总磷总氮操作日志.vi"("data in"=w425) -> ()  [unwired: 10 in, 1 out]
      }
    }
    n265 = case shown="真" w391 {
      frame False {
      }
      frame True {
        n266 = property on="多列列表框" class="MCListbox (严格)"() -> ("ItemNames"=w449:string[][], "Value"=w445:i32)  [unwired: 2 in, 2 out]
        n267 = Index Array(array=w449, index (row)=w445) -> (element=w448:string[])  [unwired: 1 in]
        n268 = Index Array(array=w448) -> (element=w447:string)  [unwired: 1 in]
        n269 = call "过滤筛选流程.vi"("字符串"=w447) -> ("匹配后偏移量"=w446:i32)  [unwired: 10 in]
        n270 = case shown="默认" w446 {
          tunnel: w447 -> [w451 _]
          tunnel: w445 -> [w450 _]
          frame Default {
            n271 = case shown="默认" w451 {
              selector: w451 -> [w457 w464]
              tunnel: [w457 w464] -> w453
              tunnel: [string[] [] ("数组") w459] -> w452
              tunnel: w450 -> [_ w463]
              frame "读数" {
              }
              frame Default {
                n272 = Equal?(x=w463, y=1) -> (x = y?=w461:bool)
                n273 = Select(t=string[] [], s=w461, f="数组") -> (s? t:f=w459:string[])
              }
            }
            n274 = for {
              N: 1 -> [_]
              tunnel: w453 -> [w466]
              shift-right: [w465] -> w454
              shift-left: w452 -> [w467]
              n275 = Search 1D Array(1D array=w467, element=w466) -> (index of element=w470:i32)  [unwired: 1 in]
              n276 = Format Into String(format string="%s" ("格式字符串"), w466) -> (resulting string=w471:string)  [unwired: 2 in, 1 out]
              n277 = Equal?(x=w470, y=-1) -> (x = y?=w468:bool)
              n278 = case shown="真" w468 {
                tunnel: w471 -> [_ w481]
                tunnel: w467 -> [w473 w485]
                tunnel: w466 -> [_ w484]
                tunnel: [w473 w483] -> w465
                frame False {
                }
                frame True {
                  n279 = Insert Into Array(array=w485, new element=w484) -> (w483:string[])  [unwired: 1 in]
                  n280 = global read "VAR总磷总氮全局变量.vi" "状态告警区"() -> (w480:T5)
                  n281 = Unbundle By Name(w480) -> ("工作状态"=w479:u16, "flowid"=w474:u16)
                  n282 = case shown="1" w479 {
                    selector: w479 -> [w500 _ _ _ _ _ _ _ _ _ _ _]
                    tunnel: [w499 "【水样测试】" ("字符串") w503 "【零点核查】" ("字符串") "【跨度核查】" ("字符串") "【空白测试】" ("字符串") "【平行样测试】" ("字符串") "【加标回收】" ("字符串") "【空白校准】" ("字符串") "【标样校准】" ("字符串") "【单步调试】" ("字符串") w514] -> w477
                    tunnel: w474 -> [_ _ w502 _ _ _ _ _ _ _ _ _]
                    frame 0, Default {
                      n283 = Number To Decimal String(number=w500) -> (decimal integer string=w499:string)  [unwired: 1 in]
                    }
                    frame 1 {
                    }
                    frame 2 {
                      n284 = case shown="默认" w502 {
                        tunnel: ["【标样核查】" ("字符串") "【快捷测试】" ("字符串")] -> w503
                        frame Default {
                        }
                        frame 5 {
                        }
                      }
                    }
                    frame 3 {
                    }
                    frame 4 {
                    }
                    frame 5 {
                    }
                    frame 6 {
                    }
                    frame 7 {
                    }
                    frame 8 {
                    }
                    frame 9 {
                    }
                    frame 254 {
                    }
                    frame 255 {
                      n285 = local read "简易步骤名称"() -> (w516:string)
                      n286 = Format Into String(format string="(%s)" ("格式字符串"), initial string="【简易流程】" ("工作状态"), w516) -> (resulting string=w514:string)  [unwired: 1 in, 1 out]
                    }
                  }
                  n287 = global read "VAR总磷总氮全局变量.vi" "状态告警区"() -> (w498:T5)
                  n288 = global read "VAR总磷总氮全局变量.vi" "状态告警区"() -> (w495:T5)
                  n289 = Unbundle By Name(w495) -> ("F0"=w492:sgl, "F1"=w491:sgl, "F2"=w490:sgl, "F3"=w489:sgl, "id"=w488:u16, "flowid"=w487:u16, "量程"=w486:u16)
                  n290 = Unbundle By Name(w498) -> ("id"=w476:u16)
                  n291 = call "id参数转换.vi"("id"=w476) -> ("table输出"=w475:string)  [unwired: 9 in, 1 out]
                  n292 = Concatenate Strings(w477, w481) -> (w478:string)
                  n293 = Format Into String(format string="F0=%#f,F1=%#f,F2=%#f,F3=%#f,Flow=%d-%-d-%-d" ("格式字符串"), w492, w491, w490, w489, w488, w487, w486) -> (resulting string=w493:string)  [unwired: 2 in, 1 out]
                  n294 = Get Date/Time In Seconds() -> (seconds since 1Jan1904=w496:timestamp)
                  n295 = Bundle By Name(cluster=T12 {"时间标识"=timestamp(0 s since 1904-01-01), "设备"="", "日志信息"="", "流程参数"=""} ("data in"), "时间标识"=w496, "设备"=w475, "日志信息"=w478, "流程参数"=w493) -> (w497:T12)
                  n296 = call "总磷总氮操作日志.vi"("data in"=w497) -> ()  [unwired: 10 in, 1 out]
                }
              }
            }
            n297 = local write "数组"(w454) -> ()
          }
          frame -1 {
          }
        }
      }
    }
    n298 = Multiply(x=w371, y=100.0) -> (x*y=w368:dbl)
    "滑动杆" <- w368
    n299 = global write "VAR总磷总氮全局变量.vi" "测试进度"(w368) -> ()
  }
  n300 = case shown="\"Bad\", 默认" w12 {
    tunnel: w11 -> [w556 w560]
    tunnel: [w556 w557] -> w10
    frame "Bad", Default {
    }
    frame "Idle" {
      n301 = invoke class="VI" method="Run VI"(reference=w560, "Wait until done"=FALSE ("结束前等待"), "Auto Dispose Ref"=TRUE ("自动销毁引用")) -> (reference out=w557:refnum<vi>)  [unwired: 2 in, 4 out]
    }
  }
  n302 = case shown="\"Bad\", 默认" w16 {
    tunnel: w15 -> [w561 w565]
    tunnel: [w561 w562] -> w14
    frame "Bad", Default {
    }
    frame "Idle" {
      n303 = invoke class="VI" method="Run VI"(reference=w565, "Wait until done"=FALSE ("结束前等待"), "Auto Dispose Ref"=TRUE ("自动销毁引用")) -> (reference out=w562:refnum<vi>)  [unwired: 2 in, 4 out]
    }
  }
  n304 = Obtain Notifier(name (unnamed)=w19, notification data type=FALSE) -> (notifier out=w20:refnum<notifier>)  [unwired: 2 in, 2 out]
  n305 = Obtain Queue(name (unnamed)=w19, element data type=cluster{"命令":string, "data":variant} {"命令"="", "data"=variant}) -> (queue out=w22:refnum<queue>)  [unwired: 3 in, 2 out]
  n306 = while {
    tunnel: w22 -> [w569]
    tunnel: w20 -> [w568]
    tunnel: w14 -> [w567]
    tunnel: w10 -> [w566]
    stop <- FALSE stop-if-true
    n307 = event shown="[7] \"停止\": 值改变" {
      selector: _ -> [_ _ _ _ _ _ _ _ _ _ _ _ _]
      dyn-events: _ -> [_ _ _ _ _ _ _ _ _ _ _ _ _]
      timeout: _ -> [_ _ _ _ _ _ _ _ _ _ _ _ _]
      tunnel: w569 -> [_ _ _ _ _ w581 _ w588 _ _ _ _ _]
      tunnel: w568 -> [_ _ _ _ _ _ _ w587 _ _ _ _ _]
      tunnel: w567 -> [_ _ _ _ _ _ _ _ w608 _ _ _ _]
      tunnel: w566 -> [_ _ _ _ _ _ _ _ _ _ _ w614 _]
      event Timeout {
        n308 = event-data() -> ()  [unwired: 1 in, 3 out]
      }
      event "温度曲线": Value Change {
        n309 = event-data() -> ()  [unwired: 1 in, 6 out]
        n310 = call "温度曲线显示.vi"() -> ()  [unwired: 12 in]
      }
      event "启动参数设置": Value Change {
        n311 = event-data() -> ()  [unwired: 1 in, 6 out]
        n312 = call "启动参数设置.vi"() -> ()  [unwired: 12 in]
      }
      event "布尔": Value Change {
        n313 = event-data() -> ("NewVal"=w571:bool)  [unwired: 1 in, 5 out]
        n314 = case shown="假" w571 {
          frame False {
            n315 = global write "VAR总磷总氮全局变量.vi" "权限等级"(enum16{"一级权限", "二级权限", "三级权限", "超级权限"}."一级权限" ("权限等级")) -> ()
          }
          frame True {
            n316 = global read "VAR总磷总氮全局变量.vi" "权限密码"() -> (w575:u32[])
            n317 = global read "VAR总磷总氮全局变量.vi" "权限等级"() -> (w573:enum16{"一级权限", "二级权限", "三级权限", "超级权限"})
            n318 = call "密码权限设置.vi"("权限输入"=w573, "权限密码"=w575) -> ("权限输出"=w574:enum16{"一级权限", "二级权限", "三级权限", "超级权限"})  [unwired: 9 in]
            n319 = global write "VAR总磷总氮全局变量.vi" "权限等级"(w574) -> ()
          }
        }
      }
      event "权限等级": Mouse Down {
        n320 = event-data() -> ()  [unwired: 1 in, 8 out]
        n321 = global read "VAR总磷总氮全局变量.vi" "权限密码"() -> (w578:u32[])
        n322 = global read "VAR总磷总氮全局变量.vi" "权限等级"() -> (w576:enum16{"一级权限", "二级权限", "三级权限", "超级权限"})
        n323 = call "密码权限设置.vi"("权限输入"=w576, "权限密码"=w578) -> ("权限输出"=w577:enum16{"一级权限", "二级权限", "三级权限", "超级权限"})  [unwired: 9 in]
        n324 = global write "VAR总磷总氮全局变量.vi" "权限等级"(w577) -> ()
      }
      event "手动启动": Value Change {
        n325 = event-data() -> ()  [unwired: 1 in, 6 out]
        n326 = call "总磷总氮启动参数对话框.vi"() -> ("确认"=w579:bool, "元素"=w580:cluster{"命令":string, "data":variant})  [unwired: 10 in]
        n327 = case shown="真" w579 {
          tunnel: w581 -> [_ w584]
          tunnel: w580 -> [_ w583]
          frame False {
          }
          frame True {
            n328 = Flush Queue(queue=w584) -> (queue out=w582:refnum<queue>)  [unwired: 1 in, 2 out]
            n329 = Enqueue Element(queue=w582, element=w583) -> ()  [unwired: 2 in, 3 out]
          }
        }
      }
      event "调试": Value Change {
        n330 = event-data() -> ()  [unwired: 1 in, 6 out]
        n331 = call "总磷单步调试对话框.vi"() -> ()  [unwired: 12 in]
      }
      event "停止": Value Change {
        n332 = event-data() -> ()  [unwired: 1 in, 6 out]
        n333 = Two Button Dialog(message="确认停止？" ("消息")) -> (T button?=w585:bool)  [unwired: 2 in]
        n334 = case shown="真" w585 {
          tunnel: w588 -> [_ w601]
          tunnel: w587 -> [_ w600]
          frame False {
          }
          frame True {
            n335 = Send Notification(notification=TRUE ("通知"), notifier=w600) -> ()  [unwired: 1 in, 2 out]
            n336 = global read "VAR总磷总氮全局变量.vi" "状态告警区"() -> (w592:T5)
            n337 = global read "VAR总磷总氮全局变量.vi" "状态告警区"() -> (w598:T5)
            n338 = Unbundle By Name(w592) -> ("id"=w591:u16)
            n339 = Unbundle By Name(w598) -> ("id"=w597:u16)
            n340 = case shown="3, 92" w597 {
              tunnel: [_ cluster{"命令":string, "data":variant} {"命令"="启动", "data"=variant(cluster{"站号":u16, "控制命令输出":u16[]} {"站号"=1, "控制命令输出"=[2816]})} ("元素") cluster{"命令":string, "data":variant} {"命令"="启动", "data"=variant(cluster{"站号":u16, "控制命令输出":u16[]} {"站号"=2, "控制命令输出"=[2816]})} ("元素") cluster{"命令":string, "data":variant} {"命令"="启动", "data"=variant(cluster{"站号":u16, "控制命令":u16[]} {"站号"=3, "控制命令"=[2816]})} ("元素")] -> w596
              frame 0, Default {
              }
              frame 1, 131 {
              }
              frame 2, 76 {
              }
              frame 3, 92 {
              }
            }
            n341 = call "id参数转换.vi"("id"=w591) -> ("table输出"=w590:string)  [unwired: 9 in, 1 out]
            n342 = Get Date/Time In Seconds() -> (seconds since 1Jan1904=w594:timestamp)
            n343 = Bundle By Name(cluster=T12 {"时间标识"=timestamp(0 s since 1904-01-01), "设备"="", "日志信息"="", "流程参数"=""} ("data in"), "时间标识"=w594, "设备"=w590, "日志信息"="手动停止") -> (w593:T12)
            n344 = call "总磷总氮操作日志.vi"("data in"=w593) -> ()  [unwired: 10 in, 1 out]
            n345 = Enqueue Element(queue=w601, element=w596) -> ()  [unwired: 2 in, 3 out]
          }
        }
      }
      event "参数设置", "参数查询": Value Change {
        n346 = event-data() -> ()  [unwired: 1 in, 6 out]
        n347 = invoke on="子面板" class="SubPnl" method="Remove VI"() -> (error out=w609:errorcluster)  [unwired: 3 in, 2 out]
        n348 = property on="仪器校准" class="Bool"("Visible"=TRUE ("可见")) -> ()  [unwired: 2 in, 2 out]
        n349 = property on="窗格" class="Pane"("Origin"=T4 {"Horizontal"=0, "Vertical"=640} ("原点")) -> ()  [unwired: 2 in, 2 out]
        n350 = property on="参数查询" class="Bool"("Visible"=FALSE ("可见")) -> ()  [unwired: 2 in, 2 out]
        n351 = global write "VAR总磷总氮全局变量.vi" "页面"(enum16{"主页", "参数页", "校准页"}."参数页" ("页面")) -> ()
        n352 = invoke on="子面板" class="SubPnl" method="Insert VI"(error in=w609, "VI Ref"=w608) -> ()  [unwired: 2 in, 4 out]
      }
      event "修改系列号": Value Change {
        n353 = event-data() -> ()  [unwired: 1 in, 6 out]
        n354 = call "写入系列号对话框.vi"() -> ()  [unwired: 12 in]
      }
      event "流程写入": Value Change {
        n355 = event-data() -> ()  [unwired: 1 in, 6 out]
        n356 = call "流程复合写入.vi"() -> ()  [unwired: 12 in]
      }
      event "仪器校准": Value Change {
        n357 = event-data() -> ()  [unwired: 1 in, 6 out]
        n358 = invoke on="子面板" class="SubPnl" method="Remove VI"() -> (error out=w615:errorcluster)  [unwired: 3 in, 2 out]
        n359 = property on="参数查询" class="Bool"("Visible"=TRUE ("可见")) -> ()  [unwired: 2 in, 2 out]
        n360 = property on="仪器校准" class="Bool"("Visible"=FALSE ("可见")) -> ()  [unwired: 2 in, 2 out]
        n361 = global write "VAR总磷总氮全局变量.vi" "页面"(enum16{"主页", "参数页", "校准页"}."校准页" ("页面")) -> ()
        n362 = invoke on="子面板" class="SubPnl" method="Insert VI"(error in=w615, "VI Ref"=w614) -> ()  [unwired: 2 in, 4 out]
      }
      event "返回": Value Change {
        n363 = event-data() -> ()  [unwired: 1 in, 6 out]
        n364 = global write "VAR总磷总氮全局变量.vi" "页面"(enum16{"主页", "参数页", "校准页"}."主页" ("页面")) -> ()
        n365 = property on="窗格" class="Pane"("Origin"=T4 {"Horizontal"=0, "Vertical"=0} ("原点")) -> ()  [unwired: 2 in, 2 out]
      }
    }
  }
  n366 = while {
    tunnel: w22 -> [w631]
    stop <- FALSE stop-if-true
    n367 = Wait (ms)(milliseconds to wait=u32 1000 ("等待时间（毫秒）")) -> ()  [unwired: 1 out]
    n368 = global read "总磷总氮断电保存全局变量.vi" "MB通信方式选择"() -> (w629:enum16{"串口", "TCP"})
    n369 = global read "VAR总磷总氮全局变量.vi" "升级固件关闭心跳包"() -> (w621:bool)
    n370 = global read "VAR总磷总氮全局变量.vi" "MB session in"() -> (w627:refnum<class "MB_Master.lvclass">)
    n371 = case shown="\"串口\", 默认" w629 {
      tunnel: [w634 w635] -> w628
      frame "串口", Default {
        n372 = global read "总磷总氮断电保存全局变量.vi" "VISA Resource"() -> (w634:refnum<visa-resource-name>)
      }
      frame "TCP" {
        n373 = global read "总磷总氮断电保存全局变量.vi" "IP"() -> (w635:string)
      }
    }
    "字符串 2" <- w628
    n374 = property class="MB_Master"(reference=w627) -> ("Properties:Session Valid"=w625:bool)  [unwired: 1 in, 2 out]
    n375 = Not(x="关闭心跳包") -> (.not. x?=w623:bool)
    n376 = Not(x=w621) -> (.not. x?=w620:bool)
    n377 = Get Queue Status(queue=w631) -> (queue out=w630:refnum<queue>, # elements in queue=w626:i32)  [unwired: 2 in, 6 out]
    n378 = Equal To 0?(x=w626) -> (x = 0?=w618:bool)
    n379 = Compound Arithmetic op=AND ("复合运算")(w625, w623, w620) -> (w622:bool)
    n380 = global write "VAR总磷总氮全局变量.vi" "心跳包打开状态"(w622) -> ()
    n381 = And(x=w622, y=w618) -> (x .and. y?=w619:bool)
    n382 = case shown="真" w619 {
      tunnel: w630 -> [_ w649]
      frame False {
      }
      frame True {
        n383 = global read "总磷总氮断电保存全局变量.vi" "启动队列名称"() -> (w638:cluster{"String":string, "Value":u16}[])
        n384 = for {
          tunnel: [w667] -> w639 mode=indexing
          tunnel: w638 -> [w668] mode=indexing
          n385 = Unbundle By Name(w668) -> ("Value"=w667:u16)
        }
        n386 = global read "VAR总磷总氮全局变量.vi" "状态告警区"() -> (w641:T5)
        n387 = Unbundle By Name(w641) -> ("系统时间"=w648:timestamp, "工作状态"=w640:u16)
        n388 = for {
          tunnel: w640 -> [w653]
          shift-right: [w654] -> w642
          shift-left: w649 -> [w656]
          tunnel: w639 -> [w650] mode=indexing
          n389 = Equal?(x=w653, y=T14."空闲") -> (x = y?=w651:bool)
          n390 = Bundle By Name(cluster=cluster{"命令":string, "data":variant} {"命令"="", "data"=variant} ("元素"), "命令"="读状态告警区", "data"=w650) -> (w658:cluster{"命令":string, "data":variant})
          n391 = Enqueue Element(queue=w656, element=w658) -> (queue out=w655:refnum<queue>)  [unwired: 2 in, 2 out]
          n392 = case shown="真" w651 {
            tunnel: w655 -> [w660 w663]
            tunnel: w650 -> [_ w662]
            tunnel: [w660 w661] -> w654
            frame False {
            }
            frame True {
              n393 = Bundle By Name(cluster=cluster{"命令":string, "data":variant} {"命令"="", "data"=variant} ("元素"), "命令"="读测量数据区", "data"=w662) -> (w665:cluster{"命令":string, "data":variant})
              n394 = Enqueue Element(queue=w663, element=w665) -> (queue out=w661:refnum<queue>)  [unwired: 2 in, 2 out]
            }
          }
        }
        n395 = Get Date/Time In Seconds() -> (seconds since 1Jan1904=w647:timestamp)
        n396 = Subtract(x=w647, y=w648) -> (x-y=w646:dbl)
        n397 = Absolute Value(x=w646) -> (abs(x)=w645:dbl)
        n398 = global read "VAR总磷总氮全局变量.vi" "通讯状态"() -> (w636:bool)
        n399 = Greater Or Equal?(x=w645, y=30.0) -> (x >= y?=w643:bool)
        n400 = And(x=w643, y=w636) -> (x .and. y?=w637:bool)
        n401 = case shown="假" w637 {
          tunnel: w642 -> [_ w676]
          tunnel: [w669 _] -> _
          frame False {
            n402 = global read "VAR总磷总氮全局变量.vi" "MB session in"() -> (w672:refnum<class "MB_Master.lvclass">)
            n403 = call "版本号读取.vi"("MB session in"=w672) -> ("error out"=w670:errorcluster, "固件版本号"=→"固件版本号":string, "MB session out"=w671:refnum<class "MB_Master.lvclass">)  [unwired: 8 in]
            n404 = call "序列号读取.vi"("Error in"=w670, "MB session in"=w671) -> ("error out"=w669:errorcluster, "序列号"=w674:string)  [unwired: 7 in, 1 out]
            n405 = global write "VAR总磷总氮全局变量.vi" "序列号"(w674) -> ()
          }
          frame True {
            n406 = call "总磷总氮启动命令.vi"("参数"=T15 {"站号"=3, "量程切换"=enum."AUTO", "控制命令"=enum."校时", "模式设置"=enum."待机", "测量间隔"=0}) -> ("启动命令"=w675:cluster{"命令":string, "data":variant})  [unwired: 10 in]
            n407 = Enqueue Element(queue=w676, element=w675) -> ()  [unwired: 2 in, 3 out]
          }
        }
      }
    }
  }
